vi "Rename Class Controls.vi"(8 "error in (no error)":errorcluster, 9 "Old Class":path, 10 "Class to Rename":refnum<vi>, 11 "App Ref":refnum<vi>) -> (0 "error out":errorcluster)   [LabVIEW 2020]
uses:
  <vilib>/Utility/traverseref.llb/TRef TravTarget.ctl
  <vilib>/Utility/traverseref.llb/VI Scripting - Traverse.lvlib
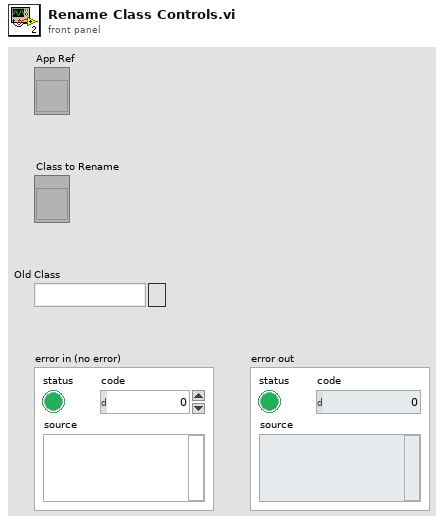
[diagram p1: front panel]
types:
  T1 = typedef "TRef TravTarget.ctl" = enum16{"FP", "BD", "Other"}
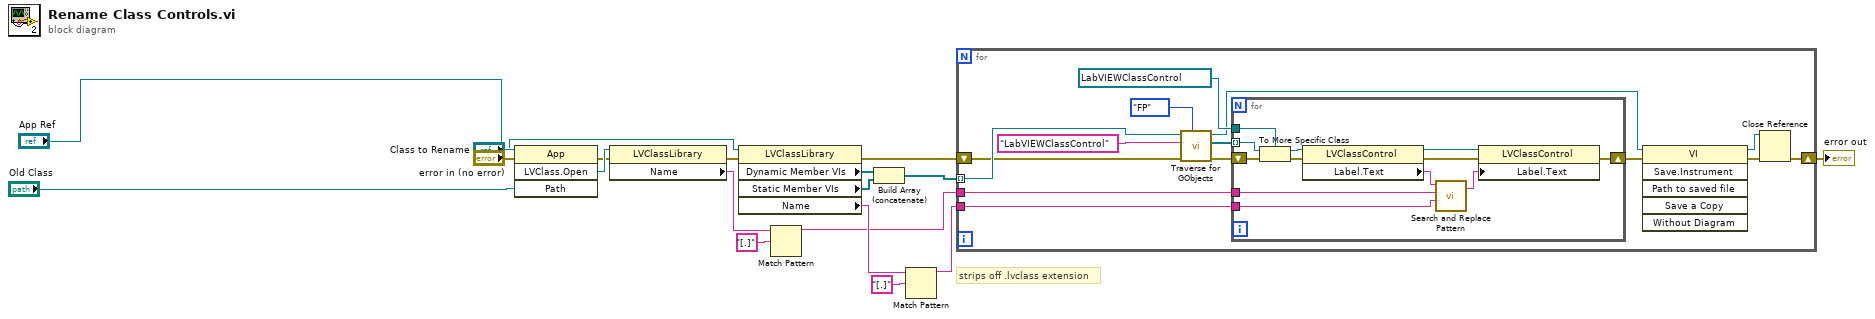
[diagram p0: block diagram]
diagram:
  # "strips off .lvclass extension"
  n1 = invoke class="App" method="LVClass.Open"(reference="App Ref", error in="error in (no error)", "Path"="Old Class") -> (error out=w15:errorcluster, "LVClass.Open"=w17:refnum<vi>)  [unwired: 1 in, 2 out]
  n2 = property class="LVClassLibrary"(reference=w17, error in=w15) -> (error out=w16:errorcluster, "Name"=w14:string)  [unwired: 1 out]
  n3 = property class="LVClassLibrary"(reference="Class to Rename", error in=w16) -> (error out=w10:errorcluster, "Dynamic Member VIs"=w4:refnum<vi>[], "Static Member VIs"=w5:refnum<vi>[], "Name"=w11:string)  [unwired: 1 out]
  n4 = Match Pattern(string=w14, regular expression="[.]") -> (before substring=w3:string)  [unwired: 1 in, 3 out]
  n5 = Build Array (concatenate)(w4, w5) -> (w6:refnum<vi>[])
  n6 = Match Pattern(string=w11, regular expression="[.]") -> (before substring=w9:string)  [unwired: 1 in, 3 out]
  n7 = for {
    tunnel: w6 -> [w32] mode=indexing
    tunnel: w9 -> [w27]
    tunnel: w3 -> [w26]
    shift-right: [w21] -> w1
    shift-left: w10 -> [w25]
    n8 = call <vilib>:"Traverse for GObjects.vi"("Traverse Target"=TRef_TravTarget."FP", "error in (no error)"=w25, "Class Name"="LabVIEWClassControl", "VI Refnum"=w32) -> ("error out"=w24:errorcluster, "References"=w29:refnum<vi>[], "dup VI Refnum"=w19:refnum<vi>)  [unwired: 4 in, 1 out]
    n9 = for {
      tunnel: w29 -> [w44] mode=indexing
      tunnel: refnum<vi> refnum ("LVClassControl Refnum") -> [w42]
      tunnel: w27 -> [w37]
      tunnel: w26 -> [w35]
      shift-right: [w33] -> w23
      shift-left: w24 -> [w34]
      n10 = To More Specific Class(target class=w42, reference=w44, error in=w34) -> (specific class reference=w43:refnum<vi>, error out=w41:errorcluster)
      n11 = property class="LVClassControl"(reference=w43, error in=w41) -> (reference out=w40:refnum<vi>, error out=w39:errorcluster, "Label.Text"=w38:string)
      n12 = call <vilib>:"Search and Replace Pattern.vi"("string"=w38, "regular expression (\"\")"=w35, "replace string (\"\")"=w37) -> ("result string"=w36:string)  [unwired: 2 in, 1 out]
      n13 = property class="LVClassControl"(reference=w40, error in=w39, "Label.Text"=w36) -> (error out=w33:errorcluster)  [unwired: 1 out]
    }
    n14 = invoke class="VI" method="Save.Instrument"(reference=w19, error in=w23) -> (reference out=w20:refnum<vi>, error out=w22:errorcluster)  [unwired: 4 in, 4 out]
    n15 = Close Reference(reference=w20, error in (no error)=w22) -> (error out=w21:errorcluster)
  }
  "error out" <- w1
